vi "RunRvp8Cal.vi"(2 "error in (no error)":errorcluster) -> (0 "error out":errorcluster)   [LabVIEW 2009]
doc: "Test out attenuation switching."
uses:
  Rvp8PowerData.ctl
panel:
  out "Frequency Ghz":dbl=2.809
  out "Cal differences":cluster{dbl[], dbl[]}[](graph)
  in  "Transfer switch":bool
  in  "Cal data directory":string="/home/operator/data"
  out "Cal output file name":string
  out "Cal  results array":string[](array[string])
  out "RVP8 calibration":cluster{dbl[], dbl[]}[](graph)
  out "RVP8_power":T1
  out "Siggen power (dBm)":dbl
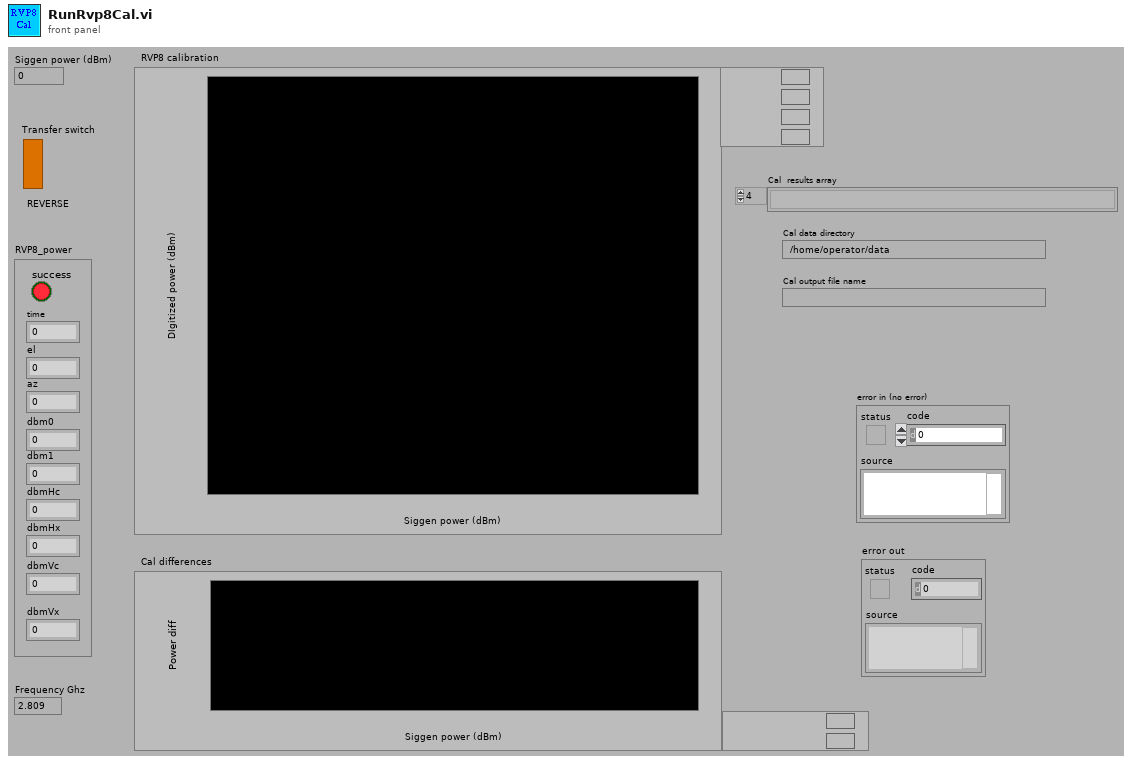
[diagram p1: front panel]
types:
  T1 = typedef "Rvp8PowerData.ctl" = cluster{"success":bool, "time":dbl, "el":dbl, "az":dbl, "dbm0":dbl, "dbm1":dbl, "dbmHc":dbl, "dbmHx":dbl, "dbmVc":dbl, "dbmVx":dbl}
  T2 = enum16{"open", "replace", "create", "open or create", "replace or create", "replace or create with confirmation"}
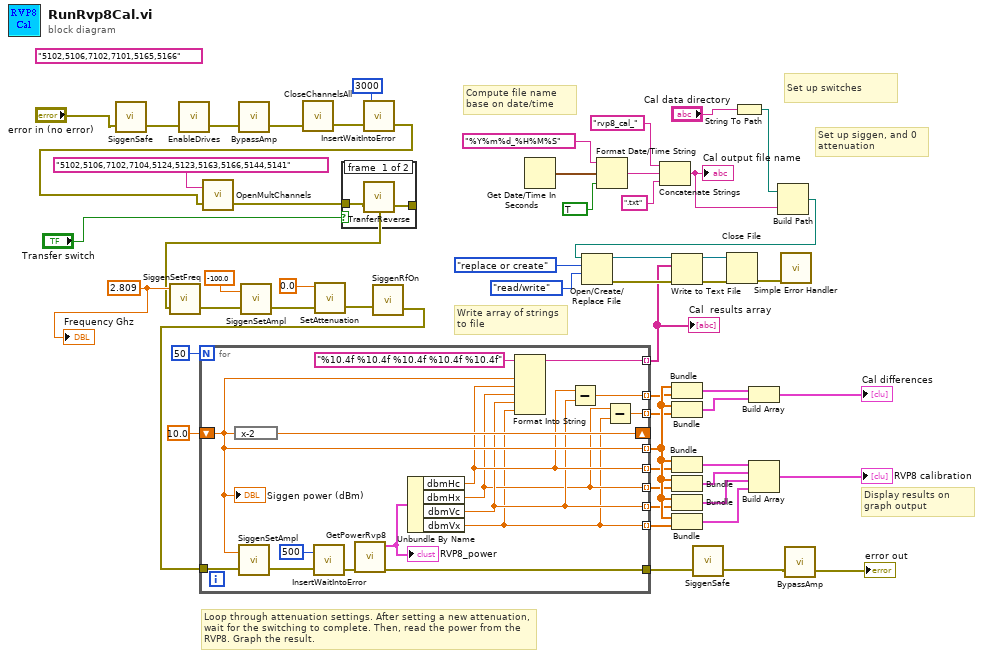
[diagram p0: block diagram]
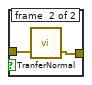
[diagram p2: hidden frame]
diagram:
  (unwired) "5102,5106,7102,7101,5165,5166"
  w55 = 2.809
  # "Set up switches"
  # "Display results on graph output"
  # "Write array of strings to file"
  # "Compute file name base on date/time"
  # "Loop through attenuation settings. After setting a new attenuation, wait for the switching to complete. Then, read the power from the RVP8. Graph the result."
  # "Set up siggen, and 0 attenuation"
  n1 = call "SiggenSafe.vi"("error in (no error)"="error in (no error)") -> ("error out"=w21:errorcluster)  [unwired: 2 in]
  n2 = call "EnableDrives.vi"("error in (no error)"=w21) -> ("error out"=w20:errorcluster)  [unwired: 2 in]
  n3 = call "BypassAmp.vi"("error in (no error)"=w20) -> ("error out"=w19:errorcluster)  [unwired: 2 in]
  n4 = call "CloseChannelsAll.vi"("error in (no error)"=w19) -> ("error out"=w49:errorcluster)  [unwired: 2 in]
  n5 = call "InsertWaitIntoError.vi"("error in (no error)"=w49, "Wait (msecs)"=3000) -> ("error out"=w11:errorcluster)  [unwired: 1 in]
  n6 = call "OpenMultChannels.vi"("error in (no error)"=w11, "Channels to be opened"="5102,5106,7102,7104,5124,5123,5163,5166,5144,5141") -> ("error out"=w9:errorcluster)  [unwired: 1 in]
  n7 = case shown="True" "Transfer switch" {
    tunnel: w9 -> [w57 w60]
    tunnel: [w58 w59] -> w8
    frame #0 {
      n8 = call "TranferReverse.vi"("error in (no error)"=w57) -> ("error out"=w58:errorcluster)  [unwired: 2 in]
    }
    frame #1 {
      n9 = call "TranferNormal.vi"("error in (no error)"=w60) -> ("error out"=w59:errorcluster)  [unwired: 2 in]
    }
  }
  n10 = call "SiggenSetFreq.vi"("error in (no error)"=w8, "Freq request (GHz)"=w55) -> ("Error status"=w17:errorcluster)  [unwired: 1 out]
  n11 = call "SiggenSetAmpl.vi"("error in (no error)"=w17, "Amplitude request (dBm)"=-100.0) -> ("error out"=w16:errorcluster)  [unwired: 1 out]
  n12 = call "SetAttenuation.vi"("error in (no error)"=w16, "Attenuation (dB)"=0.0) -> ("error out"=w18:errorcluster)  [unwired: 1 in]
  n13 = call "SiggenRfOn.vi"("error in (no error)"=w18) -> ("error out"=w7:errorcluster)  [unwired: 2 in]
  n14 = for {
    N: 50 -> [_]
    shift-right: [w67] -> _
    shift-left: 10.0 -> [w70]
    tunnel: w7 -> [w73]
    tunnel: [w76] -> w14
    tunnel: [w70] -> w56 mode=indexing
    tunnel: [w66] -> w44 mode=indexing
    tunnel: [w63] -> w43 mode=indexing
    tunnel: [w65] -> w42 mode=indexing
    tunnel: [w62] -> w41 mode=indexing
    tunnel: [w69] -> w33 mode=indexing
    tunnel: [w64] -> w6 mode=indexing
    tunnel: [w61] -> w2 mode=indexing
    n15 = expression code="x-2"(w70) -> (w67:dbl)
    n16 = call "SiggenSetAmpl.vi"("error in (no error)"=w73, "Amplitude request (dBm)"=w70) -> ("error out"=w72:errorcluster)  [unwired: 1 out]
    n17 = call "InsertWaitIntoError.vi"("error in (no error)"=w72, "Wait (msecs)"=500) -> ("error out"=w75:errorcluster)  [unwired: 1 in]
    n18 = call "GetPowerRvp8.vi"("error in (no error)"=w75) -> ("Comm error"=w76:errorcluster, "RVP8_power"=w71:T1)  [unwired: 4 in, 2 out]
    "RVP8_power" <- w71
    n19 = Unbundle By Name(w71) -> ("dbmHc"=w66:dbl, "dbmHx"=w63:dbl, "dbmVc"=w65:dbl, "dbmVx"=w62:dbl)
    n20 = Format Into String(format string="%10.4f %10.4f %10.4f %10.4f %10.4f", w70, w66, w63, w65, w62) -> (resulting string=w69:string)  [unwired: 2 in, 1 out]
    n21 = Subtract(x=w66, y=w65) -> (x-y=w64:dbl)
    n22 = Subtract(x=w63, y=w62) -> (x-y=w61:dbl)
    "Siggen power (dBm)" <- w70
  }
  "Cal  results array" <- w33
  n23 = Get Date/Time In Seconds() -> (seconds since 1Jan1904=w32:timestamp)
  n24 = Format Date/Time String(time format string (%c)="%Y%m%d_%H%M%S", seconds (now)=w32, UTC format=TRUE) -> (date/time string=w29:string)
  n25 = Concatenate Strings("rvp8_cal_", w29, ".txt") -> (w24:string)
  "Cal output file name" <- w24
  n26 = Bundle(w56, w6) -> (w4:cluster{dbl[], dbl[]})  [unwired: 1 in]
  n27 = Bundle(w56, w2) -> (w1:cluster{dbl[], dbl[]})  [unwired: 1 in]
  n28 = Bundle(w56, w44) -> (w5:cluster{dbl[], dbl[]})  [unwired: 1 in]
  n29 = Bundle(w56, w43) -> (w47:cluster{dbl[], dbl[]})  [unwired: 1 in]
  n30 = Bundle(w56, w42) -> (w46:cluster{dbl[], dbl[]})  [unwired: 1 in]
  n31 = Bundle(w56, w41) -> (w48:cluster{dbl[], dbl[]})  [unwired: 1 in]
  n32 = call "SiggenSafe.vi"("error in (no error)"=w14) -> ("error out"=w13:errorcluster)  [unwired: 2 in]
  n33 = String To Path(string="Cal data directory") -> (path=w25:path)
  n34 = Build Array(w4, w1) -> (→"Cal differences":cluster{dbl[], dbl[]}[])
  n35 = Build Array(w5, w47, w46, w48) -> (→"RVP8 calibration":cluster{dbl[], dbl[]}[])
  n36 = Build Path(base path=w25, name or relative path=w24) -> (appended path=w23:path)
  n37 = Open/Create/Replace File(file path (use dialog)=w23, operation (0:open)=T2."replace or create", access (0:read/write)=enum16{"read/write", "read-only", "write-only"}."read/write") -> (refnum out=w37:refnum<file>, error out=w35:errorcluster)  [unwired: 3 in, 1 out]
  n38 = Write to Text File(file (use dialog)=w37, text=w33, error in=w35) -> (refnum out=w36:refnum<file>, error out=w34:errorcluster)  [unwired: 1 in, 1 out]
  n39 = Close File(refnum=w36, error in=w34) -> (error out=w38:errorcluster)  [unwired: 1 out]
  n40 = call <vilib>:"Simple Error Handler.vi"("error in (no error)"=w38) -> ()  [unwired: 4 in, 5 out]
  n41 = call "BypassAmp.vi"("error in (no error)"=w13) -> ("error out"=→"error out":errorcluster)  [unwired: 2 in]
  "Frequency Ghz" <- w55
